vi "subAxisState.vi"(1 "AxisId":i32=1 min=1 max=9, 2 "Index":i32=1) -> ()   [LabVIEW 2020]
panel:
  in  "High":bool
  in  "Low":bool
  out "AmpOK":bool caption="power amplifier is activated"
  out "RefReady":bool caption="valid reference run is done"
  in  "Set":bool
  out "Error state":i32
  out "Axis state":i32
  out "Move state":i32
  in  "Close":bool
  # "Axis"
  # "State"
  # "Power amplifier"
  # "Current level"
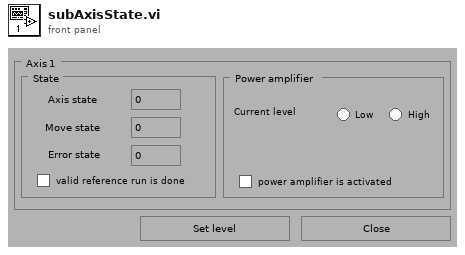
[diagram p1: front panel]
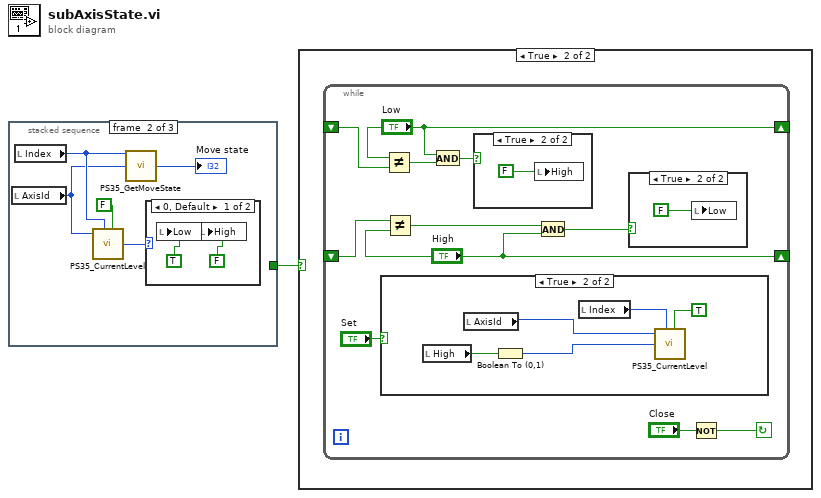
[diagram p0: block diagram]
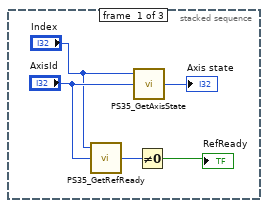
[diagram p2: hidden frame]
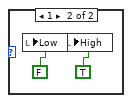
[diagram p3: hidden frame]
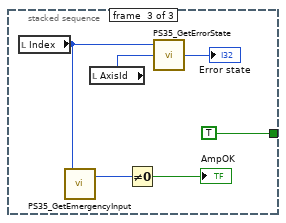
[diagram p4: hidden frame]
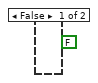
[diagram p5: hidden frame]
diagram:
  n1 = stacked-sequence {
    tunnel: [_ _ TRUE] -> w1
    frame #0 {
      n2 = call "PS35_GetRefReady.vi"("Axis number"="AxisId", "Control unit ID"="Index") -> ("State"=w5:i32)  [unwired: 2 in, 1 out]
      n3 = call "PS35_GetAxisState.vi"("Axis number"="AxisId", "Control unit ID"="Index") -> ("Axis state"=→"Axis state":i32)  [unwired: 2 in, 1 out]
      n4 = Not Equal To 0?(x=w5) -> (x != 0?=→"RefReady":bool)
    }
    frame #1 {
      n5 = local read "AxisId"() -> (w7:i32)
      n6 = local read "Index"() -> (w8:i32)
      n7 = call "PS35_CurrentLevel.vi"("Axis number"=w7, "Control unit ID"=w8, "function"=FALSE) -> ("Value-Out"=w9:i32)  [unwired: 5 in, 1 out]
      n8 = call "PS35_GetMoveState.vi"("Axis number"=w7, "Control unit ID"=w8) -> ("Move state"=→"Move state":i32)  [unwired: 2 in, 1 out]
      n9 = case shown="0, Default" w9 {
        frame 0, Default {
          n10 = local write "Low"(TRUE ("function")) -> ()
          n11 = local write "High"(FALSE ("function")) -> ()
        }
        frame 1 {
          n12 = local write "Low"(FALSE ("function")) -> ()
          n13 = local write "High"(TRUE ("function")) -> ()
        }
      }
    }
    frame #2 {
      n14 = local read "Index"() -> (w16:i32)
      n15 = call "PS35_GetEmergencyInput.vi"("Control unit ID"=w16) -> ("Value-Out"=w19:i32)  [unwired: 1 in, 1 out]
      n16 = local read "AxisId"() -> (w17:i32)
      n17 = Not Equal To 0?(x=w19) -> (x != 0?=→"AmpOK":bool)
      n18 = call "PS35_GetErrorState.vi"("Axis number"=w17, "Control unit ID"=w16) -> ("Error state"=→"Error state":i32)  [unwired: 2 in, 1 out]
    }
  }
  n19 = case shown="True" w1 {
    frame False {
      (unwired) FALSE ("End")
    }
    frame True {
      n20 = while {
        shift-left: _ -> [w29]
        shift-right: ["High"] -> _
        shift-left: _ -> [w24]
        shift-right: ["Low"] -> _
        stop <- w31 continue-if-true
        n21 = case shown="True" "Set" {
          frame False {
          }
          frame True {
            n22 = local read "High"() -> (w39:bool)
            n23 = local read "AxisId"() -> (w37:i32)
            n24 = Boolean To (0,1)(Boolean=w39) -> (0, 1=w38:i16)
            n25 = local read "Index"() -> (w35:i32)
            n26 = call "PS35_CurrentLevel.vi"("Axis number"=w37, "Control unit ID"=w35, "Value-In"=w38, "function"=TRUE) -> ()  [unwired: 4 in, 2 out]
          }
        }
        n27 = Not Equal?(x="Low", y=w24) -> (x != y?=w25:bool)
        n28 = Not Equal?(x=w29, y="High") -> (x != y?=w28:bool)
        n29 = And(x="Low", y=w25) -> (x .and. y?=w26:bool)
        n30 = case shown="True" w26 {
          frame False {
          }
          frame True {
            n31 = local write "High"(FALSE ("function")) -> ()
          }
        }
        n32 = And(x=w28, y="High") -> (x .and. y?=w27:bool)
        n33 = case shown="True" w27 {
          frame False {
          }
          frame True {
            n34 = local write "Low"(FALSE ("function")) -> ()
          }
        }
        n35 = Not(x="Close") -> (.not. x?=w31:bool)
      }
    }
  }
